vi "Compute Sweep Duration.vi"(0 "FM Sweep in":refnum<class "FM Sweep.lvclass">, 11 "error in (no error)":errorcluster) -> (4 "FM Sweep out":refnum<class "FM Sweep.lvclass">, 8 "Duration (ms)":dbl, 15 "error out":errorcluster)   [LabVIEW 2015, in "FM Sweep.lvclass"]
uses:
  FM Sweep.lvclass
  FM Sweep.lvclass/FM Sweep.ctl
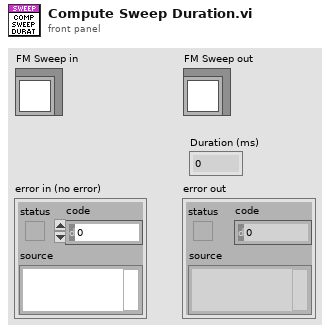
[diagram p1: front panel]
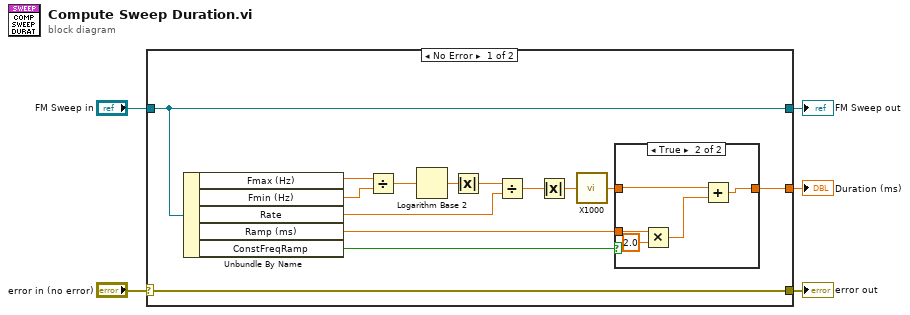
[diagram p0: block diagram]
diagram:
  n1 = case shown="No Error" "error in (no error)" {
    selector: "error in (no error)" -> [w19 w27]
    tunnel: [w19 w27] -> w4
    tunnel: [w17 w26] -> w2
    tunnel: "FM Sweep in" -> [w17 w26]
    tunnel: [w7 _] -> w1
    frame No Error {
      n2 = Unbundle By Name(w17) -> ("Fmax (Hz)"=w18:dbl, "Fmin (Hz)"=w16:dbl, "Rate"=w13:dbl, "Ramp (ms)"=w8:dbl, "ConstFreqRamp"=w9:bool)
      n3 = Divide(x=w18, y=w16) -> (x/y=w15:dbl)
      n4 = Logarithm Base 2(1:w15) -> (0:w14:dbl)
      n5 = Absolute Value(x=w14) -> (abs(x)=w6:dbl)
      n6 = Divide(x=w6, y=w13) -> (x/y=w12:dbl)
      n7 = Absolute Value(x=w12) -> (abs(x)=w11:dbl)
      n8 = call "X1000.vi"("X"=w11) -> ("X/1000"=w10:dbl)
      n9 = case shown="True" w9 {
        tunnel: w10 -> [w20 w23]
        tunnel: w8 -> [_ w25]
        tunnel: [w20 w21] -> w7
        frame False {
        }
        frame True {
          n10 = Multiply(x=w25, y=2.0) -> (x*y=w22:dbl)
          n11 = Add(x=w23, y=w22) -> (x+y=w21:dbl)
        }
      }
    }
    frame Error {
    }
  }
  "error out" <- w4
  "FM Sweep out" <- w2
  "Duration (ms)" <- w1
